vi "split flat hierarchy.vi"(8 "error in":errorcluster, 10 "UID":string, 11 "flat hierarchy":T1) -> (0 "error out":errorcluster, 2 "flat hierarchy with UID":T1, 3 "flat hierarchy without UID":T1)   [LabVIEW 2023, in "CEF.lvlib"]
doc: "Splits a hierarchy of flattened data at a given instance ID. The first output contains the original tree without the instance specified or any of its children. The second output contains the specified instance and all children, with the specified instance as the new root.Copyright 2017 National Instruments Corporation\n\nLicensed under the Apache License, Version 2.0 (the \"License\"); you may not use this file except in compliance with the License. You may obtain a copy of the License at http://www.apache.org/licenses/LICENSE-2.0\nUnless required by applicable law or agreed to in writing, software distributed under the License is distributed on an \"AS IS\" BASIS, WITHOUT WARRANTIES OR CONDITIONS OF ANY KIND, either express or implied. See the License for the specific language governing permissions and limitations under the License."
uses:
  CEF.lvlib
  hierarchy element.ctl
  instance data.ctl
  flat hierarchy.ctl
  hierarchy repo/full hierarchy.ctl
  hierarchy repo/CEF_HierarchyRepo.lvclass
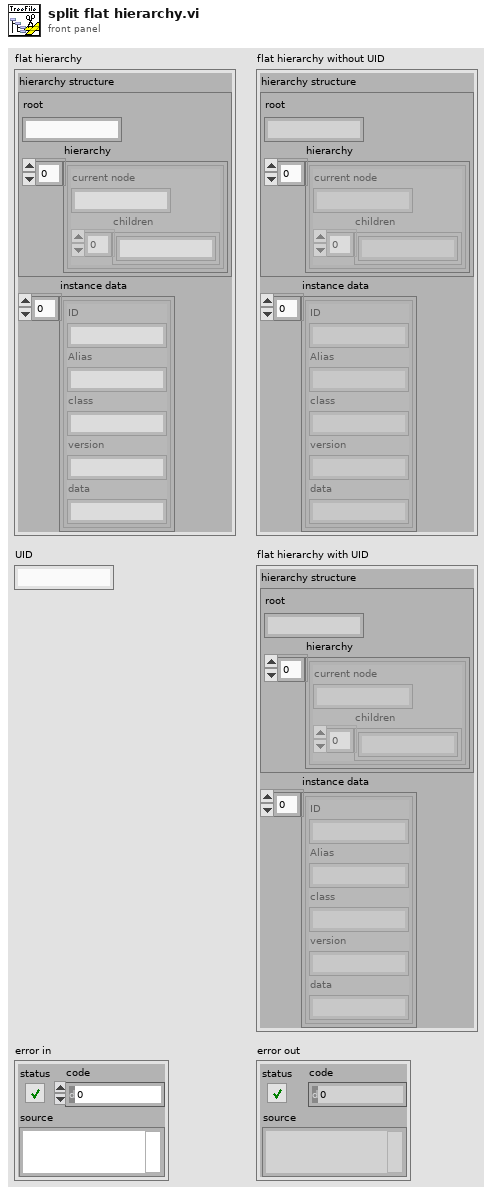
[diagram p1: front panel]
types:
  T1 = typedef "CEF.lvlib/flat hierarchy.ctl" = cluster{"hierarchy structure":T2, "instance data":T4[]}
  T2 = typedef "CEF.lvlib/CEF_HierarchyRepo.lvclass/full hierarchy.ctl" = cluster{"root":string, "hierarchy":T3[]}
  T3 = typedef "CEF.lvlib/hierarchy element.ctl" = cluster{"current node":string, "children":string[]}
  T4 = typedef "CEF.lvlib/instance data.ctl" = cluster{"ID":string, "Alias":string, "class":string, "version":string, "data":string}
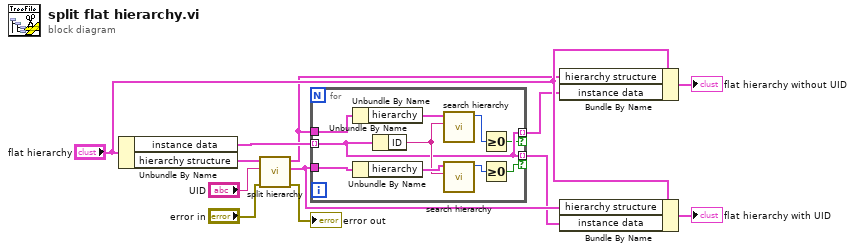
[diagram p0: block diagram]
diagram:
  n1 = Unbundle By Name("flat hierarchy") -> ("instance data"=w6:T4[], "hierarchy structure"=w12:T2)
  n2 = call "split hierarchy.vi"("error in"="error in", "UID to split"="UID", "hierarchy structure"=w12) -> ("error out"=→"error out":errorcluster, "hierarchy containing UID"=w4:T2, "hierarchy excluding UID"=w5:T2)  [unwired: 5 in, 1 out]
  n3 = for {
    tunnel: w6 -> [w17] mode=indexing
    tunnel: w5 -> [w22]
    tunnel: w4 -> [w21]
    tunnel: [w17] -> w2 mode=indexing if=w13
    tunnel: [w17] -> w3 mode=indexing if=w14
    n4 = Unbundle By Name(w22) -> ("hierarchy"=w18:T3[])
    n5 = Unbundle By Name(w21) -> ("hierarchy"=w20:T3[])
    n6 = Unbundle By Name(w17) -> ("ID"=w19:string)
    n7 = call "search hierarchy.vi"("ID"=w19, "hierarchy"=w18) -> ("index"=w16:i32)  [unwired: 9 in]
    n8 = call "search hierarchy.vi"("ID"=w19, "hierarchy"=w20) -> ("index"=w15:i32)  [unwired: 9 in]
    n9 = Greater Or Equal To 0?(x=w16) -> (x >= 0?=w13:bool)
    n10 = Greater Or Equal To 0?(x=w15) -> (x >= 0?=w14:bool)
  }
  n11 = Bundle By Name(cluster="flat hierarchy", "hierarchy structure"=w5, "instance data"=w2) -> (→"flat hierarchy without UID":T1)
  n12 = Bundle By Name(cluster="flat hierarchy", "hierarchy structure"=w4, "instance data"=w3) -> (→"flat hierarchy with UID":T1)
